vi "Steering Frame Caller.vi"() -> (3 "steering frame":refnum<class "NI_Robotics_Steering Frame.lvclass">)   [LabVIEW 2017, in "NI_Robotics_Create Steering Frame.xnode"]
uses:
  <vilib>/robotics/Steering/Create Steering Frame/NI_Robotics_Create Steering Frame.xnode
  <vilib>/robotics/Steering/Steering Frame/NI_Robotics_Steering Frame.lvclass
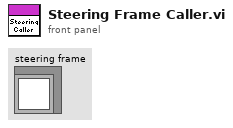
[diagram p1: front panel]
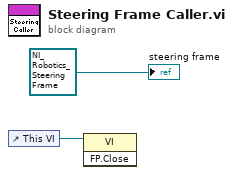
[diagram p0: block diagram]
diagram:
  n1 = control-ref of="This VI"() -> (w2:refnum<vi>)
  n2 = invoke class="VI" method="FP.Close"(reference=w2) -> ()  [unwired: 2 in, 3 out]
  "steering frame" <- refnum<class "NI_Robotics_Steering Frame.lvclass"> refnum ("NI_Robotics_Steering Frame.lvclass")
